vi "ReadValByRefNamedTxtVal.vi"(0 "Control Ref":refnum<vi>, 2 "Type In":enum16{""}(ring), 11 "error in":errorcluster caption="entrée d'erreur") -> (4 "Valeur":string, 15 "error out":errorcluster caption="sortie d'erreur")   [LabVIEW 2019]
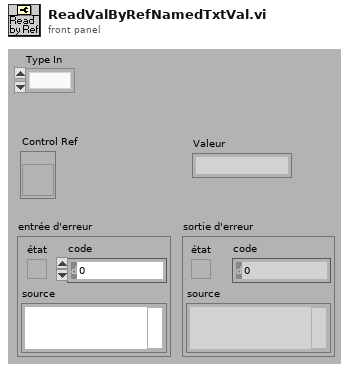
[diagram p1: front panel]
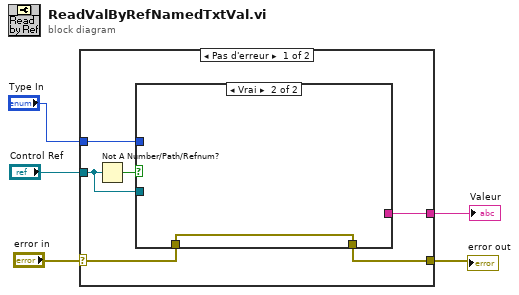
[diagram p0: block diagram]
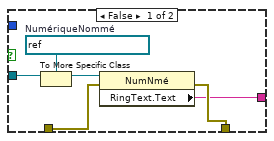
[diagram p2: hidden frame]
diagram:
  n1 = case shown="Pas d'erreur" "error in" {
    selector: "error in" -> [w9 w19]
    tunnel: "Control Ref" -> [w10 _]
    tunnel: [w8 w19] -> w3
    tunnel: "Type In" -> [w7 _]
    tunnel: [w6 _] -> w1
    frame No Error {
      n2 = Not A Number/Path/Refnum?(number/path/refnum=w10) -> (NaN/Path/Refnum?=w11:bool)
      n3 = case shown="Vrai" w11 {
        tunnel: w10 -> [w15 _]
        tunnel: [w14 _] -> w6
        tunnel: w9 -> [w17 w18]
        tunnel: [w16 w18] -> w8
        tunnel: w7 -> [_ _]
        frame False {
          w12 = refnum<vi> refnum  # NumériqueNommé
          n4 = To More Specific Class(target class=w12, reference=w15) -> (specific class reference=w13:refnum<vi>)  [unwired: 1 in, 1 out]
          n5 = property class="NumNmé"(reference=w13, error in=w17) -> (error out=w16:errorcluster, "RingText.Text"=w14:string)  [unwired: 1 out]
        }
        frame True {
        }
      }
    }
    frame Error {
    }
  }
  "Valeur" <- w1
  "error out" <- w3
